vi "viByteArrayToSI16Array4CAN.vi"(1 "input variable":u8[](array[numeric])) -> (0 "output variable":i16[](array[numeric]))   [LabVIEW 2011]
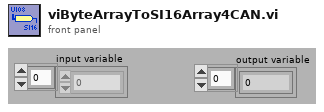
[diagram p1: front panel]
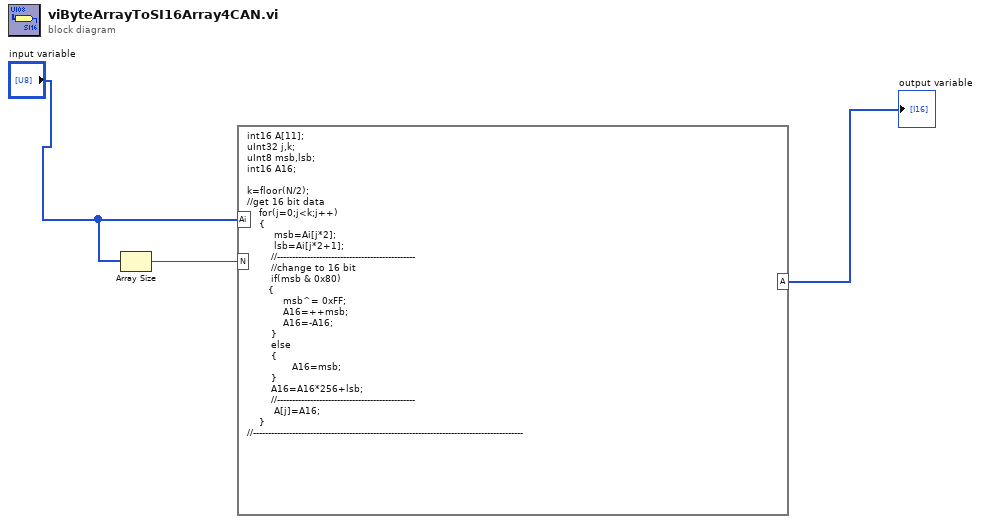
[diagram p0: block diagram]
diagram:
  n1 = Array Size(array="input variable") -> (size(s)=w3:i32)
  n2 = formula code="int16 A[11];\nuInt32 j,k;\nuInt8 msb,lsb; \nint16 A16;\n\nk=floor(N/2);\n//get 16 bit data\n    for(j=0;j<k;j++)\n    {\n         msb=Ai[j*2];\n         lsb=Ai[j*2+1];\n        //----------------------------------------------\n        //change to 16 bit      \n        if(msb & 0x80)\n       {\n            msb^= 0xFF; \n            A16=++msb;\n            A16=-A16;\n        }\n        else\n        {\n               A16=msb;\n        }\n        A16=A16*256+lsb;\n        //----------------------------------------------\n         A[j]=A16;\n    }\n//------------------------------------------------------------------------------------------"("Ai"="input variable", "N"=w3) -> ("A"=→"output variable":i16[])
